vi "ASM.StatePreAction.vi"(8 "error in (no error)":errorcluster, 11 "AsmTestMachine in":refnum<class "AsmTestMachine.lvclass">) -> (0 "error out":errorcluster, 3 "AsmTestMachine out":refnum<class "AsmTestMachine.lvclass">)   [LabVIEW 2021, in "AsmTestMachine.lvlib" / "AsmTestMachine.lvclass"]
uses:
  AsmTestMachine.lvclass
  D:/_uliarczj/_sandbox/SWTest/Utilities/LabVIEW/ActorStateMachine/Source/ActorStateMachine/ActorStateMachine/ActorStateMachine.lvclass
  AsmTestMachine.lvclass/AsmTestMachine.ctl
  Source/ActorStateMachine/ActorStateMachine/ActorStateMachine.lvclass/ActorStateMachine.ctl
  Source/ActorStateMachine/ActorStateMachine/Read CurrentState.vi
  Source/ActorStateMachine/ActorStateMachine/ActorStateMachine.lvclass
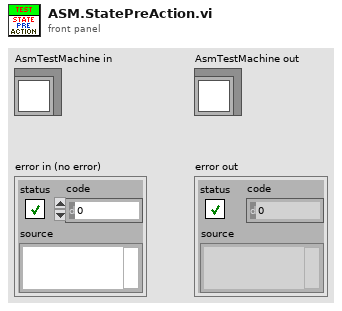
[diagram p1: front panel]
types:
  T1 = typedef "ActorStateMachine.lvlib/ActorStateMachine.lvclass/_ASM.State.ctl" = enum16{"Boom", "Pre-Init", "Init", "Post-Init", "Pre-Reset", "Reset", "Post-Reset", "Pre-Config", "Config", "Post-Config", "Pre-Ready", "Ready", "Post-Ready", "Pre-Running", "Running", "Next", "Post-Running", "Break", "Fail", "Crash", "Shutdown", "Doom"}
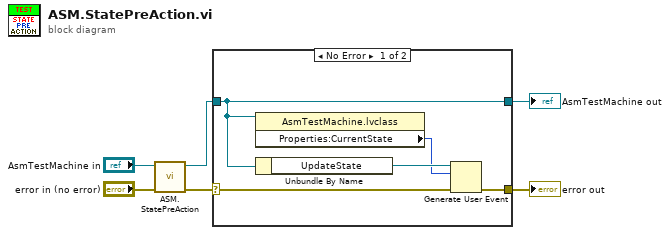
[diagram p0: block diagram]
diagram:
  n1 = call-parent "ASM.StatePreAction.vi"("error in (no error)"="error in (no error)", "ActorStateMachine in"="AsmTestMachine in") -> ("error out"=w3:errorcluster, "ActorStateMachine out"=w1:refnum<class "AsmTestMachine.lvclass">)  [unwired: 8 in]
  n2 = case shown="No Error" w3 {
    selector: w3 -> [w8 w13]
    tunnel: [w7 w13] -> w6
    tunnel: [w10 w12] -> w5
    tunnel: w1 -> [w10 w12]
    frame No Error {
      n3 = property class="AsmTestMachine.lvclass"(reference=w10) -> ("Properties:CurrentState"=w9:T1)  [unwired: 1 in, 2 out]
      n4 = Unbundle By Name(w10) -> ("UpdateState"=w11:refnum<user-event>)
      n5 = Generate User Event(user event=w11, event data cluster=w9, error in=w8) -> (error out=w7:errorcluster)  [unwired: 1 in, 1 out]
    }
    frame Error {
    }
  }
  "error out" <- w6
  "AsmTestMachine out" <- w5
